vi "Convert2RegInt32ToInt32.vi"() -> ()   [LabVIEW 2019]
panel:
  out "Hex LowWord":i32 format="%x"
  out "Result Or [Dec]":i32
  out "cast Hex manuel":i32 format="%x"
  out "cast Hex":i32 format="%x"
  in  "Input":i32
  out "Result Hex":i32 format="%x"
  out "Result if Low neg  [Dec]":i32
  out "2^16 Hex":i32 format="%x"
  in  "stop":bool
  out "Result Cast  [Dec]":i32
  out "HighWord":i16
  out "LowWord":i16
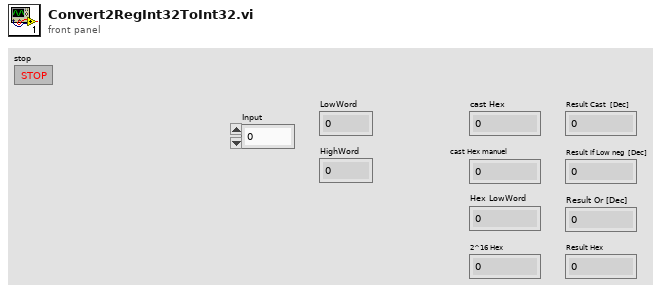
[diagram p1: front panel]
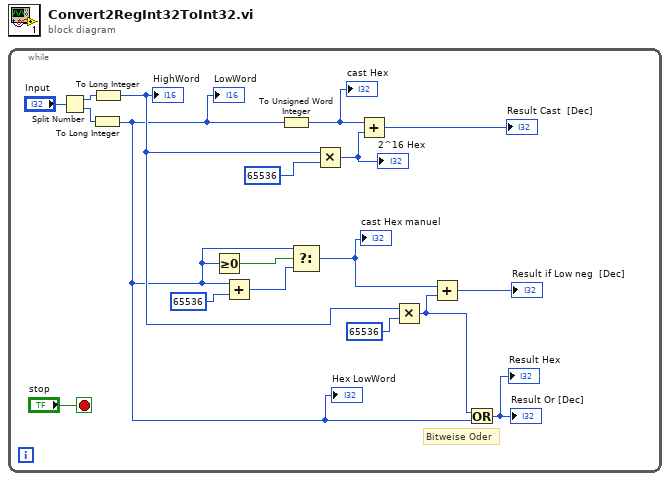
[diagram p0: block diagram]
diagram:
  n1 = while {
    stop <- "stop" stop-if-true
    # "Bitweise Oder"
    n2 = Split Number(x="Input") -> (hi(x)=w12:u16, lo(x)=w11:u16)
    n3 = To Long Integer(number=w11) -> (32bit integer=w1:i32)
    "LowWord" <- w1
    "Hex LowWord" <- w1
    n4 = To Long Integer(number=w12) -> (32bit integer=w4:i32)
    "HighWord" <- w4
    n5 = Greater Or Equal To 0?(x=w1) -> (x >= 0?=w7:bool)
    n6 = Add(x=w1, y=65536) -> (x+y=w6:i32)
    n7 = To Unsigned Word Integer(number=w1) -> (unsigned 16bit integer=w10:u16)
    "cast Hex" <- w10
    n8 = Select(t=w1, s=w7, f=w6) -> (s? t:f=w5:i32)
    "cast Hex manuel" <- w5
    n9 = Multiply(x=w4, y=65536) -> (x*y=w15:i32)
    "2^16 Hex" <- w15
    n10 = Add(x=w10, y=w15) -> (x+y=→"Result Cast  [Dec]":i32)
    n11 = Multiply(x=w4, y=65536) -> (x*y=w3:i32)
    n12 = Add(x=w5, y=w3) -> (x+y=→"Result if Low neg  [Dec]":i32)
    n13 = Or(x=w3, y=w1) -> (x .or. y?=→"Result Hex" →"Result Or [Dec]":i32)
  }
